vi "Add Version Values.vi"(8 "error in (no error)":errorcluster, 10 "Version":T1, 11 "Map in":map{string, string}(c390)) -> (0 "error out":errorcluster, 3 "Map out":map{string, string}(c390))   [LabVIEW 2019, in "NIPKG Packager.lvclass"]
uses:
  NIPKG Packager.lvclass
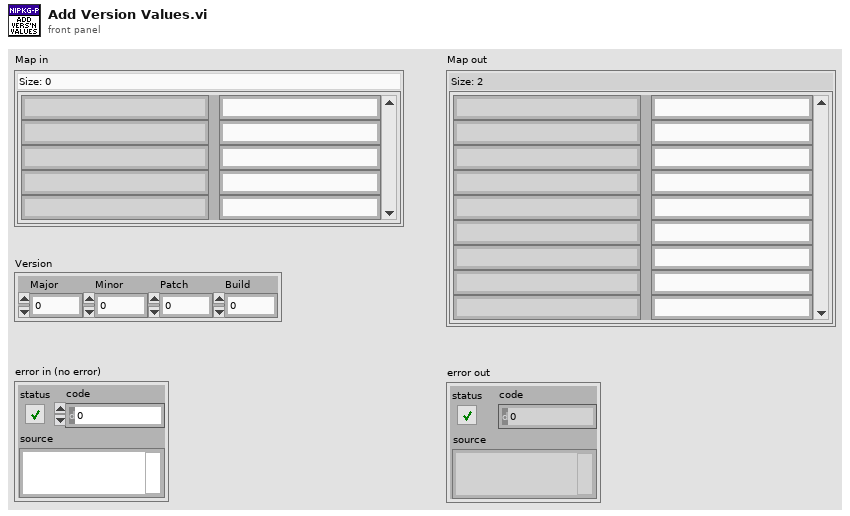
[diagram p1: front panel]
types:
  T1 = cluster{"Major":i32, "Minor":i32, "Patch":i32, "Build":i32}
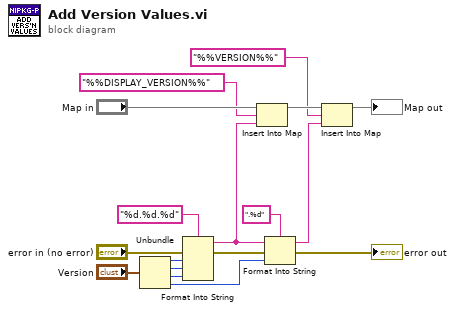
[diagram p0: block diagram]
diagram:
  n1 = Unbundle("Version") -> ("Major"=w4:i32, "Minor"=w3:i32, "Patch"=w1:i32, "Build"=w2:i32)
  n2 = Format Into String(format string="%d.%d.%d", error in="error in (no error)", w4, w3, w1) -> (resulting string=w9:string, error out=w13:errorcluster)  [unwired: 1 in]
  n3 = Insert Into Map(map in="Map in", key="%%DISPLAY_VERSION%%", value=w9) -> (map out=w17:map{string, string})  [unwired: 2 out]
  n4 = Format Into String(format string=".%d", initial string=w9, error in=w13, w2) -> (resulting string=w6:string, error out=→"error out":errorcluster)
  n5 = Insert Into Map(map in=w17, key="%%VERSION%%", value=w6) -> (map out=→"Map out":map{string, string})  [unwired: 2 out]
